vi "Detect Steering Misalignment.vi"(11 "Motors In":T1 {"Radii (ft)"."Right Back Position" format="%.2f"; "Radii (ft)"."Right Front Position" format="%.2f"; "Radii (ft)"."Left Back Position" format="%.2f"; "Radii (ft)"."Left Front Position" format="%.2f"; "Pigeon2"."Type" items=["CAN"=352321536, "TalonSRX"=33554432]}) -> (3 "Motors Out":T1 {"Radii (ft)"."Right Back Position" format="%.2f"; "Radii (ft)"."Right Front Position" format="%.2f"; "Radii (ft)"."Left Back Position" format="%.2f"; "Radii (ft)"."Left Front Position" format="%.2f"; "Pigeon2"."Type" items=["CAN"=352321536, "TalonSRX"=33554432]})   [LabVIEW 2023]
uses:
  swerve/Type Definitions/Hardware/Swerve Drives/(NEO-NEO-ThroughBore-Pigeon2) Swerve.ctl
  swerve/Type Definitions/Hardware/4 Motor Sets/(NEO & NEO 550) 4 Motor Set.ctl
  <vilib>/Rock Robotics/WPI/MotorControl/WPI_MotorControlDeviceRef.ctl
  <vilib>/Rock Robotics/WPI/MotorControl/WPI_MotorControlType.ctl
  <vilib>/Rock Robotics/SystemInterfaces/DIO/FPGA_DIOPWMChannel.ctl
  <vilib>/Rock Robotics/WPI/PWM/WPI_PWMDeadband.ctl
  <vilib>/Rock Robotics/SystemInterfaces/DIO/FPGA_DIOChannel.ctl
  <vilib>/Rock Robotics/WPI/ThirdParty/Phoenix-LabVIEW/Pigeon IMU/CTRE_PigeonIMU_DeviceRef.ctl
  <vilib>/Rock Robotics/WPI/ThirdParty/Phoenix-LabVIEW/Pigeon IMU/CTRE_PigeonIMU_ConnectionType.ctl
  swerve/Type Definitions/Data/Pod Positions.ctl
  <vilib>/Analysis/coordinate.llb/Angle Units.ctl
  5e800f26-b426-49e4-b681-eb18440e8622.vi
  <vilib>/Analysis/coordinate.llb/Wrap Angle (scalar).vi
  <vilib>/Rock Robotics/WPI/ThirdParty/REV Robotics/REVLib/SubVI/Public/SPARK Get Absolute Encoder Status Position.vi
  <vilib>/Rock Robotics/Network Tables/NT Read String.vi
  <vilib>/Analysis/NI_AAL_Angle.lvlib
types:
  T1 = typedef "(NEO-NEO-ThroughBore-Pigeon2) Swerve.ctl" = cluster{"Drive Motors (NEO)":T2, "Steer Motors (NEO)":T2, "Pigeon2":T8, "Radii (ft)":T10}
  T2 = typedef "(NEO & NEO 550) 4 Motor Set.ctl" = cluster{"Left Front":T3, "Left Back":T3, "Right Front":T3, "Right Back":T3}
  T3 = typedef "WPI_MotorControlDeviceRef.ctl" = cluster{"DeviceStatus":errorcluster, "Type":T4, "PWM":cluster{"PWM Channel":T5, "DeadBand":T6}, "CAN":cluster{"Device Number":u8, "SetOutput VI Ref":variant, "GetOutput VI Ref":variant, "Enable VI Ref":variant, "Disable VI Ref":variant, "Data":variant}, "Invert":bool, "DIO PWM":cluster{"PWM \"Enable\" Channel":T5, "DIOChannel":T7, "PWM Rate":dbl}}
  T4 = typedef "WPI_MotorControlType.ctl" = enum16{"PWM", "CAN", "DIO PWM"}
  T5 = typedef "FPGA_DIOPWMChannel.ctl" = enum8{"PWM 0", "PWM 1", "PWM 2", "PWM 3", "PWM 4", "PWM 5", "PWM 6", "PWM 7", "PWM 8", "PWM 9", "PWM MXP 0", "PWM MXP 1", "PWM MXP 2", "PWM MXP 3", "PWM MXP 4", "PWM MXP 5", "PWM MXP 6", "PWM MXP 7", "PWM MXP 8", "PWM MXP 9", "Invalid"}
  T6 = typedef "WPI_PWMDeadband.ctl" = cluster{"Name":string, "maxPositivePwm":i32, "minPositivePwm":i32, "centerPwm":i32, "maxNegativePwm":i32, "minNegativePwm":i32, "angularRange":u16}
  T7 = typedef "FPGA_DIOChannel.ctl" = enum8{"DIO 0", "DIO 1", "DIO 2", "DIO 3", "DIO 4", "DIO 5", "DIO 6", "DIO 7", "DIO 8", "DIO 9", "DIO MXP 0", "DIO MXP 1", "DIO MXP 2", "DIO MXP 3", "DIO MXP 4", "DIO MXP 5", "DIO MXP 6", "DIO MXP 7", "DIO MXP 8", "DIO MXP 9", "DIO MXP 10", "DIO MXP 11", "DIO MXP 12", "DIO MXP 13", "DIO MXP 14", "DIO MXP 15", "SPI Port CS1", "SPI Port CS2", "SPI Port CS3", "SPI Port MISO", "SPI Port MOSI", "Invalid"}
  T8 = typedef "CTRE_PigeonIMU_DeviceRef.ctl" = cluster{"DeviceStatus":errorcluster, "Device Number":u8, "Type":T9, "Device ID":u32, "Handle":u64, "UsageFrame":u32, "Library Path":path}
  T9 = typedef "CTRE_PigeonIMU_ConnectionType.ctl" = u32
  T10 = typedef "Pod Positions.ctl" = cluster{"Left Front Position":dbl[], "Left Back Position":dbl[], "Right Front Position":dbl[], "Right Back Position":dbl[]}
  T11 = typedef "NI_AAL_Angle.lvlib/Angle Units.ctl" = i32
  T12 = cluster{"Left Front":dbl, "Left Back":dbl, "Right Front":dbl, "Right Back":dbl}
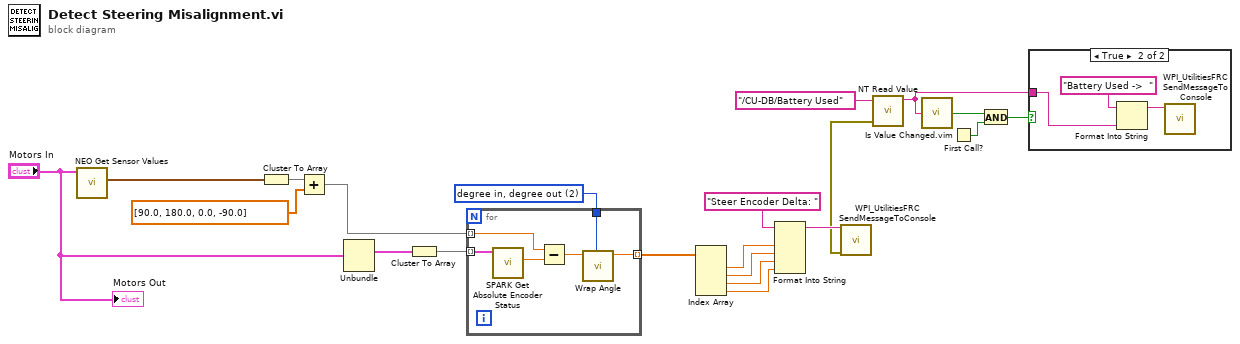
[diagram p0: block diagram]
diagram:
  w21 = T11 2 items=["radian in, radian out", "radian in, degree out", "degree in, degree out", "degree in, radian out"] ("angle units")
  n1 = call "NEO Get Sensor Values.vi"("Swerve Motors"="Motors In") -> ("Steer Angles (degrees)"=w15:T12)  [unwired: 9 in, 1 out]
  n2 = Cluster To Array(cluster=w15) -> (array=w18:dbl[])
  n3 = Add(x=w18, y=dbl[] [90.0, 180.0, 0.0, -90.0]) -> (x+y=w16:dbl[])
  n4 = Unbundle("Motors In") -> ("Steer Motors (NEO)"=w19:T2)  [unwired: 3 out]
  n5 = Cluster To Array(cluster=w19) -> (array=w20:T3[])
  n6 = for {
    tunnel: w20 -> [w27] mode=indexing
    tunnel: w16 -> [w25] mode=indexing
    tunnel: w21 -> [w23]
    tunnel: [w22] -> w7 mode=indexing
    n7 = call-poly <vilib>:"SPARK Get Absolute Encoder Status.vi"("MotorControlDeviceRef in"=w27) -> ("Position"=w26:dbl)  [unwired: 7 in, 3 out]
    n8 = Subtract(x=w25, y=w26) -> (x-y=w24:dbl)
    n9 = call-poly <vilib>:"Wrap Angle.vi"("angle units"=w23, "angle in"=w24) -> ("angle out"=w22:dbl)  [unwired: 8 in, 1 out]
  }
  n10 = Index Array(array=w7) -> (element #1=w11:dbl, element #2=w10:dbl, element #3=w9:dbl, element #4=w8:dbl)  [unwired: 4 in]
  n11 = Format Into String(initial string="Steer Encoder Delta: ", w11, w10, w9, w8) -> (resulting string=w13:string)  [unwired: 2 in, 1 out]
  n12 = call-poly <vilib>:"NT Read Value.vi"("name"="/CU-DB/Battery Used") -> ("error out"=w4:errorcluster, "value"=w5:string)  [unwired: 8 in, 1 out]
  n13 = call <vilib>:"WPI_UtilitiesFRC SendMessageToConsole.vi"("Message"=w13, "error in (no error)"=w4) -> ()  [unwired: 13 in, 1 out]
  n14 = call "Is Value Changed.vim"("value"=w5) -> ("changed or first call?"=w3:bool)
  n15 = First Call?() -> (First Call?: T/F=w1:bool)
  n16 = And(x=w3, y=w1) -> (x .and. y?=w2:bool)
  n17 = case shown="True" w2 {
    tunnel: w5 -> [_ w28]
    frame False {
    }
    frame True {
      n18 = Format Into String(initial string="Battery Used ->  ", w28) -> (resulting string=w30:string)  [unwired: 2 in, 1 out]
      n19 = call <vilib>:"WPI_UtilitiesFRC SendMessageToConsole.vi"("Message"=w30) -> ()  [unwired: 14 in, 1 out]
    }
  }
  "Motors Out" <- "Motors In"
